vi "MTS_AddFileToWorkspace.vi"(0 "File Name":path, 1 "File Type":T2(ring), 2 "Scan Axis":enum32{"x-y", "x-z", "y-x", "y-z", "z-x", "z-y"}(ring), 3 "Measurement Type":T1(ring)=enum."Image File", 5 "File Info":T3, 11 "error in (no error)":errorcluster, 12 "Parent":i32=-1, 13 "Tree Refnum":refnum<vi>) -> (4 "File Name (dup)":path, 14 "File No":i32, 15 "error out":errorcluster)   [LabVIEW 2013]
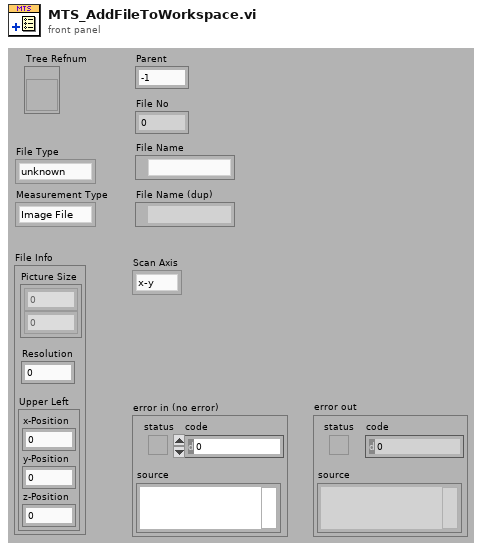
[diagram p1: front panel]
types:
  T1 = enum16{"not a pt3 File", "Image File", "Point Measurement", "Auto Point", "Line Scan", "Grid Scan"}
  T2 = enum16{"unknown", "pt3 File", "png Image", "bmp Image"}
  T3 = cluster{"Picture Size":dbl[], "Resolution":dbl, "Upper Left":cluster{"x-Position":dbl, "y-Position":dbl, "z-Position":dbl}}
  T4 = enum16{"Get (Default)", "Set Workspace", "Append File", "Change Comment"}
  T5 = cluster{"File No":i32, "File Path":path, "Parent File":i32, "File Type":enum16{"unknown", "pt3 File", "png Image", "bmp Image"}, "Measurement Type":enum16{"not a pt3 File", "Image File", "Point Measurement", "Auto Point", "Line Scan", "Grid Scan"}, "Upper Left":cluster{"x-Position":dbl, "y-Position":dbl, "z-Position":dbl}, "Pixels":i32[], "Scan Axis":enum32{"x-y", "x-z", "y-x", "y-z", "z-x", "z-y"}, "Resolution":dbl, dbl}
  T6 = cluster{"x-Position":dbl, "y-Position":dbl, "z-Position":dbl}
  T7 = cluster{"File No":i32, "File Path":path, "Parent File":i32, "File Type":enum16{"unknown", "pt3 File", "png Image", "bmp Image"}, "Measurement Type":enum16{"not a pt3 File", "Image File", "Point Measurement", "Auto Point", "Line Scan", "Grid Scan"}, "Upper Left":cluster{"x-Position":dbl, "y-Position":dbl, "z-Position":dbl}, "Pixels":i32[], "Scan Axis":enum32{"x-y", "x-z", "y-x", "y-z", "z-x", "z-y"}, "Resolution":dbl, "PixelTime":dbl}[]
  T8 = cluster{"File No":i32, "File Path":path, "Parent File":i32, "File Type":enum16{"unknown", "pt3 File", "png Image", "bmp Image"}, "Measurement Type":enum16{"not a pt3 File", "Image File", "Point Measurement", "Auto Point", "Line Scan", "Grid Scan"}, "Upper Left":cluster{"x-Position":dbl, "y-Position":dbl, "z-Position":dbl}, "Pixels":i32[], "Scan Axis":enum32{"x-y", "x-z", "y-x", "y-z", "z-x", "z-y"}, "Resolution":dbl, dbl}[]
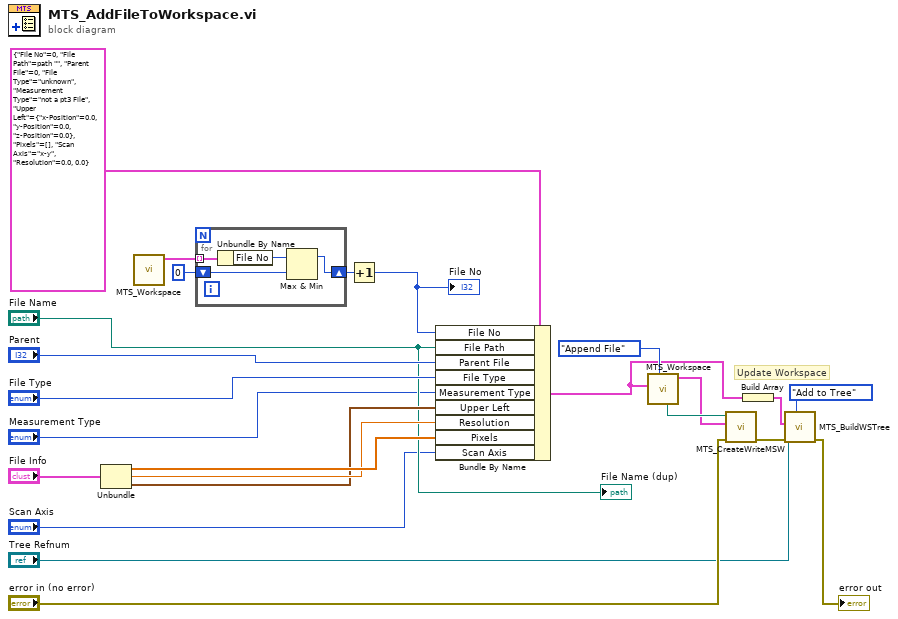
[diagram p0: block diagram]
diagram:
  # "Update Workspace"
  n1 = Unbundle("File Info") -> ("Picture Size"=w18:dbl[], "Resolution"=w17:dbl, "Upper Left"=w16:T6)
  n2 = call "MTS_Workspace.vi"() -> ("Files in Workspace"=w23:T7)  [unwired: 8 in, 3 out]
  n3 = for {
    tunnel: w23 -> [w28] mode=indexing
    shift-right: [w25] -> w21
    shift-left: 0 ("y") -> [w26]
    n4 = Unbundle By Name(w28) -> ("File No"=w27:i32)
    n5 = Max & Min(x=w27, y=w26) -> (max(x,y)=w25:i32)  [unwired: 1 out]
  }
  n6 = Increment(x=w21) -> (x+1=w20:i32)
  "File No" <- w20
  n7 = Bundle By Name(cluster=T5 {"File No"=0, "File Path"=path "", "Parent File"=0, "File Type"=enum."unknown", "Measurement Type"=enum."not a pt3 File", "Upper Left"={"x-Position"=0.0, "y-Position"=0.0, "z-Position"=0.0}, "Pixels"=[], "Scan Axis"=enum."x-y", "Resolution"=0.0, 0.0} ("Append File"), "File No"=w20, "File Path"="File Name", "Parent File"="Parent", "File Type"="File Type", "Measurement Type"="Measurement Type", "Upper Left"=w16, "Resolution"=w17, "Pixels"=w18, "Scan Axis"="Scan Axis") -> (w6:T5)
  n8 = call "MTS_Workspace.vi"("Operation"=T4."Append File", "Append File"=w6) -> ("Files in Workspace"=w2:T7, "Workspace (dup)"=w10:path)  [unwired: 6 in, 2 out]
  n9 = call "MTS_CreateWriteMSW.vi"("error in (no error)"="error in (no error)", "Files in Workspace"=w2, "Workspace Path"=w10) -> ("error out"=w9:errorcluster)  [unwired: 5 in, 3 out]
  n10 = Build Array(w6) -> (w5:T8)
  n11 = call "MTS_BuildWSTree.vi"("Action"=enum16{"Rebuild Tree", "Add to Tree"}."Add to Tree", "error in"=w9, "Files in Workspace"=w5, "Tree Refnum"="Tree Refnum") -> ("error out"=→"error out":errorcluster)  [unwired: 5 in, 2 out]
  "File Name (dup)" <- "File Name"
